vi "TLC Geometry - Stack.vi"() -> ()   [LabVIEW 2023]
doc: "This example shows how to use the 'Stack Horizontally' and 'Stack Vertically' VIs to stack objects in these two directions."
uses:
  Ctrls/alignment.ctl
  <vilib>/numeric/Random Number (Range) U64.vi
  <vilib>/numeric/sub_Random U32.vi
panel:
  in  "alignment":T1=enum."AlignLeft"
  in  "spacing[pixels]":u16
  in  "useControlBodyOnly":bool=TRUE caption="Use Ctrl Body Only\n(=ignore labels \n& captions)"
  in  "stop":bool
  in  "stackHorizontally":bool
  in  "stackVertically":bool
  in  "shuffle":bool
  in  "control 3":string
  in  "control 2":bool
  in  "control 1":string
  in  "control 0":dbl
  # "Instruction:\n1. Press the Shuffle button to place the target objects randomly.\n\n2. Press your preferred Stack button.\n\nOptional: You can also configure the horizontal alignment for vertical stacking or the vertical alignment for horizontal stacking. Additionally, you can choose to consider the control body only and adjust the spacing between objects."
  # "Stack objects"
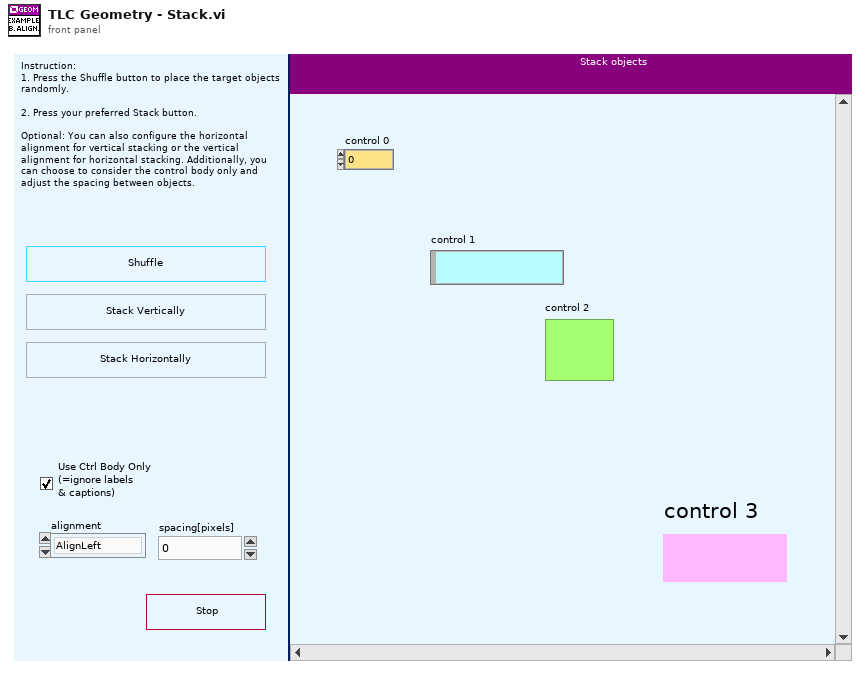
[diagram p1: front panel]
types:
  T1 = typedef "alignment.ctl" = enum16{"None", "AlignTop", "AlignBottom", "AlignHorizontalCenters", "AlignLeft", "AlignRight", "AlignVerticalCenters"}
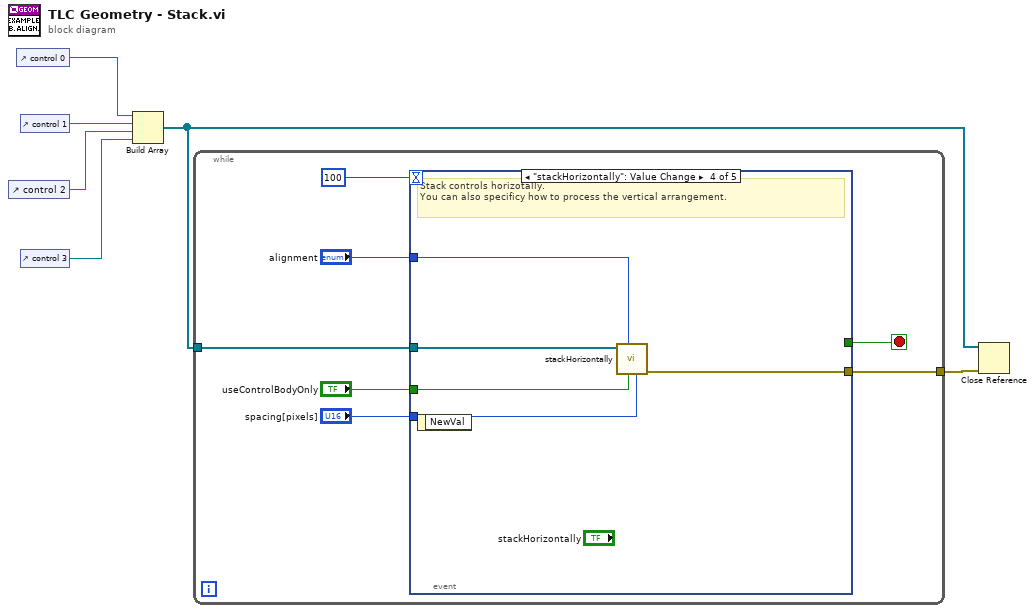
[diagram p0: block diagram]
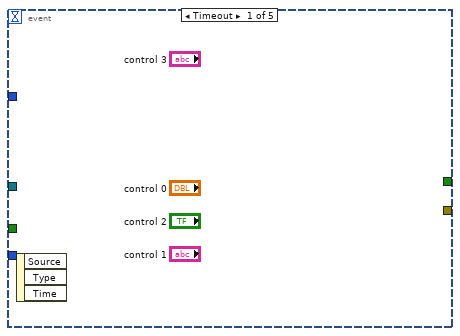
[diagram p2: hidden frame]
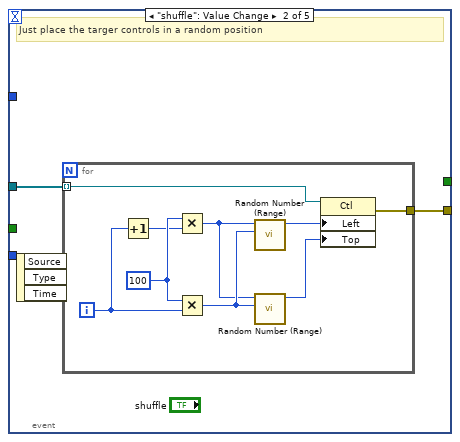
[diagram p3: hidden frame]
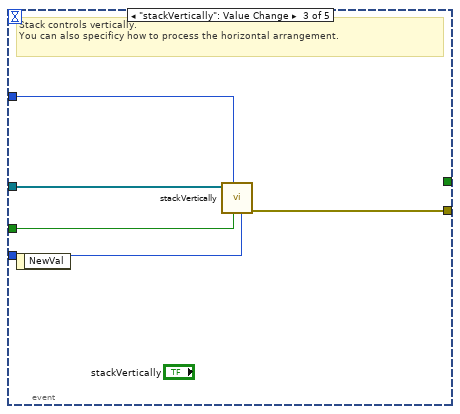
[diagram p4: hidden frame]
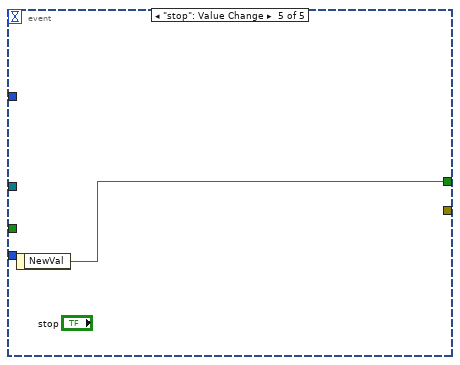
[diagram p5: hidden frame]
diagram:
  n1 = control-ref of="control 2"() -> (w5:refnum<vi>)
  n2 = control-ref of="control 0"() -> (w1:refnum<vi>)
  n3 = control-ref of="control 1"() -> (w6:refnum<vi>)
  n4 = control-ref of="control 3"() -> (w4:refnum<vi>)
  n5 = Build Array(w1, w6, w5, w4) -> (w3:refnum<vi>[])
  n6 = while {
    tunnel: w3 -> [w12]
    tunnel: [w11] -> w2
    stop <- w13 stop-if-true
    n7 = event shown="[3] \"stackHorizontally\": Value Change" {
      selector: _ -> [_ _ _ _ _]
      dyn-events: _ -> [_ _ _ _ _]
      timeout: 100 -> [_ _ _ _ _]
      tunnel: [_ _ _ _ w35] -> w13
      tunnel: w12 -> [_ w15 w29 w34 _]
      tunnel: [_ w14 w27 w32 _] -> w11
      tunnel: "useControlBodyOnly" -> [_ _ w28 w33 _]
      tunnel: "spacing[pixels]" -> [_ _ w26 w31 _]
      tunnel: "alignment" -> [_ _ w25 w30 _]
      event Timeout {
        n8 = event-data() -> ()  [unwired: 1 in, 3 out]
      }
      event "shuffle": Value Change {
        # "Just place the targer controls in a random position"
        n9 = event-data() -> ()  [unwired: 1 in, 3 out]
        n10 = for {
          tunnel: w15 -> [w24] mode=indexing
          tunnel: [w21] -> w14
          i -> [w20]
          w19 = u64 100 ("upper bound (100)")
          n11 = Increment(x=w20) -> (x+1=w17:i32)
          n12 = Multiply(x=w19, y=w17) -> (x*y=w16:u64)
          n13 = Multiply(x=w19, y=w20) -> (x*y=w18:u64)
          n14 = call-poly <vilib>:"Random Number (Range).vi"("lower bound (0)"=w18, "upper bound (100)"=w16) -> ("number"=w23:u64)  [unwired: 9 in]
          n15 = call-poly <vilib>:"Random Number (Range).vi"("lower bound (0)"=w18, "upper bound (100)"=w16) -> ("number"=w22:u64)  [unwired: 9 in]
          n16 = property class="Ctl"(reference=w24, "Left"=w23, "Top"=w22) -> (error out=w21:errorcluster)  [unwired: 1 in, 1 out]
        }
      }
      event "stackVertically": Value Change {
        # "Stack controls vertically. \nYou can also specificy how to process the horizontal arrangement."
        n17 = event-data() -> ()  [unwired: 1 in, 1 out]
        n18 = call "stackVertically.vi"("spacing[pixel]"=w26, "useControlBodyOnly"=w28, "horizontalAlignment"=w25, "refs"=w29) -> ("error out"=w27:errorcluster)  [unwired: 6 in, 1 out]
      }
      event "stackHorizontally": Value Change {
        # "Stack controls horizotally. \nYou can also specificy how to process the vertical arrangement."
        n19 = event-data() -> ()  [unwired: 1 in, 1 out]
        n20 = call "stackHorizontally.vi"("spacing[pixel]"=w31, "useControlBodyOnly"=w33, "verticalAlignment"=w30, "refs"=w34) -> ("error out"=w32:errorcluster)  [unwired: 6 in, 1 out]
      }
      event "stop": Value Change {
        n21 = event-data() -> ("NewVal"=w35:bool)  [unwired: 1 in]
      }
    }
  }
  n22 = Close Reference(reference=w3, error in (no error)=w2) -> ()  [unwired: 1 out]
